vi "HART_Write command to 973MVD.vi"(6 "data":u8[](array[numeric]), 8 "error in":errorcluster, 9 "READ Command":u8, 10 "address (array)":u8[](array[numeric]), 11 "resource name":refnum<visa-resource-name>) -> (0 "error out":errorcluster, 2 "appended array":u8[](array[numeric]) format="%x")   [LabVIEW 2016]
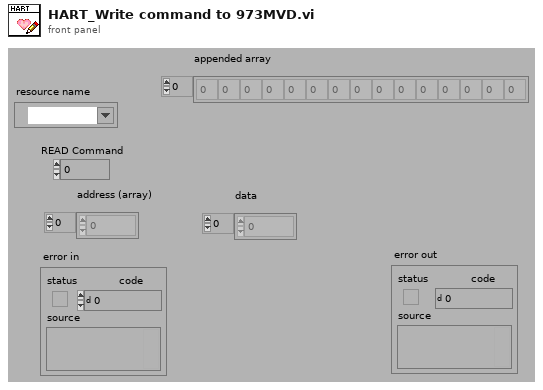
[diagram p1: front panel]
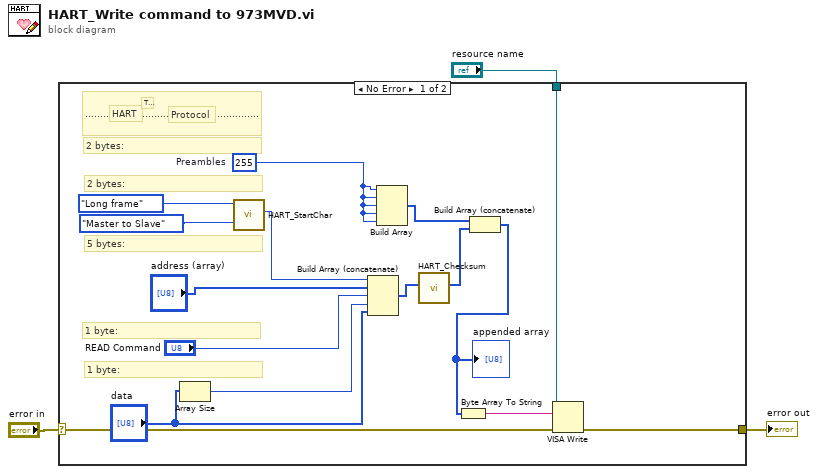
[diagram p0: block diagram]
diagram:
  n1 = case shown="No Error" "error in" {
    selector: "error in" -> [w15 w20]
    tunnel: [w17 w20] -> w3
    tunnel: "resource name" -> [w14 _]
    frame No Error {
      w10 = u8 255  # Preambles
      # "1 byte:"
      # "1 byte:"
      # "5 bytes:"
      # "2 bytes:"
      # "2 bytes:"
      # "Protocol"
      # "TM"
      # "HART"
      # ".........................................................."
      n2 = Array Size(array="data") -> (size(s)=w4:i32)
      n3 = call "HART_StartChar.vi"("Message type"=enum16{"Master to Slave", "Slave to Master"}."Master to Slave", "Address type"=enum16{"Short frame", "Long frame"}."Long frame") -> ("start character"=w13:u8)  [unwired: 9 in]
      n4 = Build Array (concatenate)(w13, "address (array)", "READ Command", w4, "data") -> (w11:i32[])
      n5 = Build Array(w10, w10, w10, w10, w10) -> (w9:u8[])
      n6 = call "HART_Checksum.vi"("message"=w11) -> ("message + chk"=w8:u8[])  [unwired: 9 in, 1 out]
      n7 = Build Array (concatenate)(w9, w8) -> (w7:u8[])
      "appended array" <- w7
      n8 = Byte Array To String(unsigned byte array=w7) -> (string=w16:string)
      n9 = VISA Write(VISA resource name=w14, write buffer=w16, error in (no error)=w15) -> (error out=w17:errorcluster)  [unwired: 2 out]
    }
    frame Error {
    }
  }
  "error out" <- w3
